vi "(auto) Get State (SubVI).vi"(8 "Dots in total":i32, 9 "States in total":i32, 10 "CurDot":T1(ring), 11 "Dots of States":i32[][](array[numeric])) -> (3 "(auto) States":T1(ring))   [LabVIEW 2017]
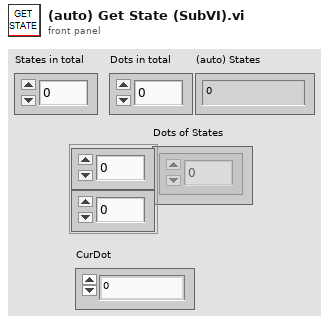
[diagram p1: front panel]
types:
  T1 = enum16{"0", "1", "2", "3", "4", "5", "6", "7", "8", "9", "10", "11", "12", "13", "14", "15", "16", "17", "18", "19", "20", "21", "22", "23", "24", "25", "26", "27", "28", "29", "30", "31", "32", "33", "34", "35"}
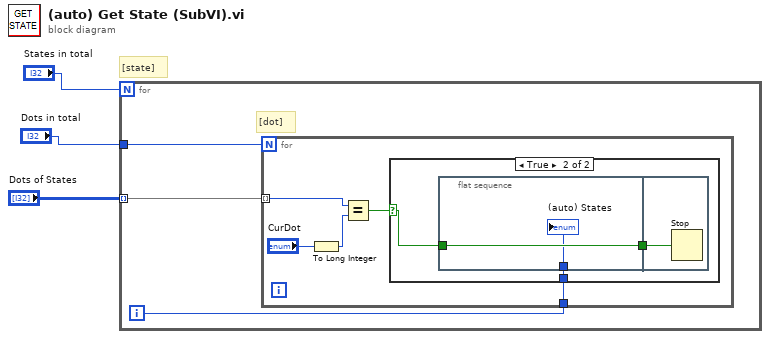
[diagram p0: block diagram]
diagram:
  # "[state]"
  n1 = for {
    N: "States in total" -> [_]
    tunnel: "Dots in total" -> [w6]
    tunnel: "Dots of States" -> [w5] mode=indexing
    i -> [w4]
    # "[dot]"
    n2 = for {
      N: w6 -> [_]
      tunnel: w5 -> [w11] mode=indexing
      tunnel: w4 -> [w7]
      n3 = To Long Integer(number="CurDot") -> (32bit integer=w9:i32)
      n4 = Equal?(x=w11, y=w9) -> (x = y?=w8:bool)
      n5 = case shown="True" w8 {
        selector: w8 -> [_ w14]
        tunnel: w7 -> [_ w12]
        frame False {
        }
        frame True {
          n6 = flat-sequence {
            tunnel: w14 -> [w16]
            tunnel: [w16] -> w13
            tunnel: w12 -> [w15]
            tunnel: w13 -> [w17]
            frame #0 {
              "(auto) States" <- w15
            }
            frame #1 {
              n7 = Stop(stop? (T)=w17) -> ()
            }
          }
        }
      }
    }
  }
